vi "Random Times.vi"(0 "Number of Interruptions":i32, 5 "Start Second":dbl format="%#_13g", 7 "Longest Gap":dbl=1.4 format="%#_13g", 9 "Shortest Gap":dbl=1.0 format="%#_13g", 11 "Error In":errorcluster) -> (4 "Interruption TImes":dbl[](array[numeric]), 15 "Error Out":errorcluster)   [LabVIEW 2020, in "CollectionSupport.lvlib"]
uses:
  CollectionSupport.lvlib
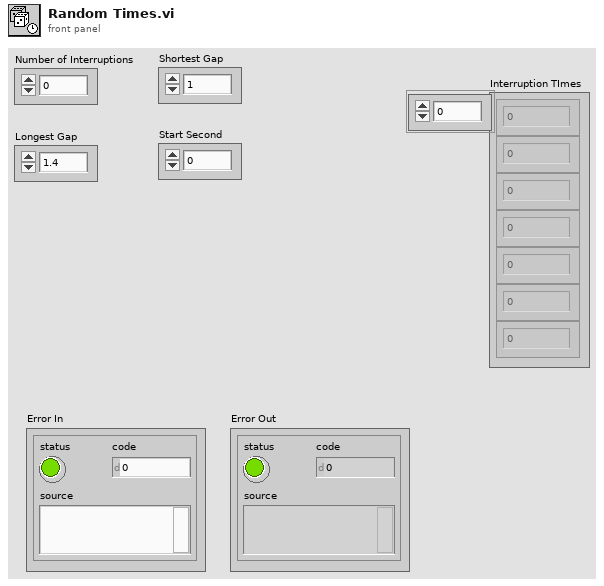
[diagram p1: front panel]
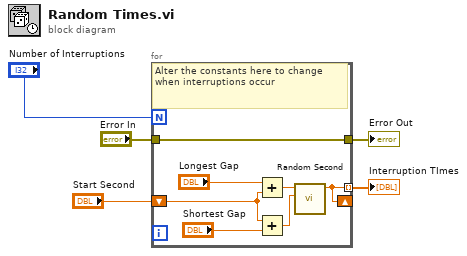
[diagram p0: block diagram]
diagram:
  n1 = for {
    N: "Number of Interruptions" -> [_]
    tunnel: [w12] -> w5 mode=indexing
    shift-right: [w12] -> _
    shift-left: "Start Second" -> [w8]
    tunnel: "Error In" -> [w9]
    tunnel: [w9] -> w1
    # "Alter the constants here to change when interruptions occur"
    n2 = Add(x="Longest Gap", y=w8) -> (x+y=w11:dbl)
    n3 = Add(x=w8, y="Shortest Gap") -> (x+y=w7:dbl)
    n4 = call "Random Second.vi"("Min Second"=w7, "Max Second"=w11) -> ("Random Second"=w12:dbl)  [unwired: 9 in]
  }
  "Error Out" <- w1
  "Interruption TImes" <- w5
